vi "Recherche Station FM.vi"() -> ()   [LabVIEW 2013]
uses:
  <vilib>/measure/NI_MAPro.lvlib
  <instrlib>/niUSRP/niUSRP Fetch Rx Data (CDB WDT).vi
  <vilib>/measure/maspectr.llb/FFT Power Spectrum and PSD for 1 Chan (CDB).vi
panel:
  in  "averaging parameters":T1={"averaging mode"=enum."Peak hold", "weighting mode"=enum."Exponential", "number of averages"=10}
  out "IQ Plot":waveform(dbl)[](graph)
  in  "Stop Button":bool
  out "Frequency Plot":cluster{"f0":dbl, "df":dbl, "magnitude":dbl[]}(graph)
  in  "device names":refnum<k15>="192.168.10.2"
  in  "active antenna":string="RX2"
  in  "timeout":dbl=10.0
  in  "number of samples":i64=10000
  out "error out":errorcluster
  out "coerced gain":dbl=10.0 format="%#_6f"
  out "coerced carrier frequency":dbl=315000000.0 format="%#_6p"
  out "coerced IQ rate":dbl=5000000.0 format="%#_6p"
  in  "gain":dbl=10.0 format="%#_6f"
  in  "carrier frequency":dbl=100000000.0 format="%#_6p"
  in  "IQ rate":dbl=4000000.0 format="%#_6p"
  # "IQ Receiver"
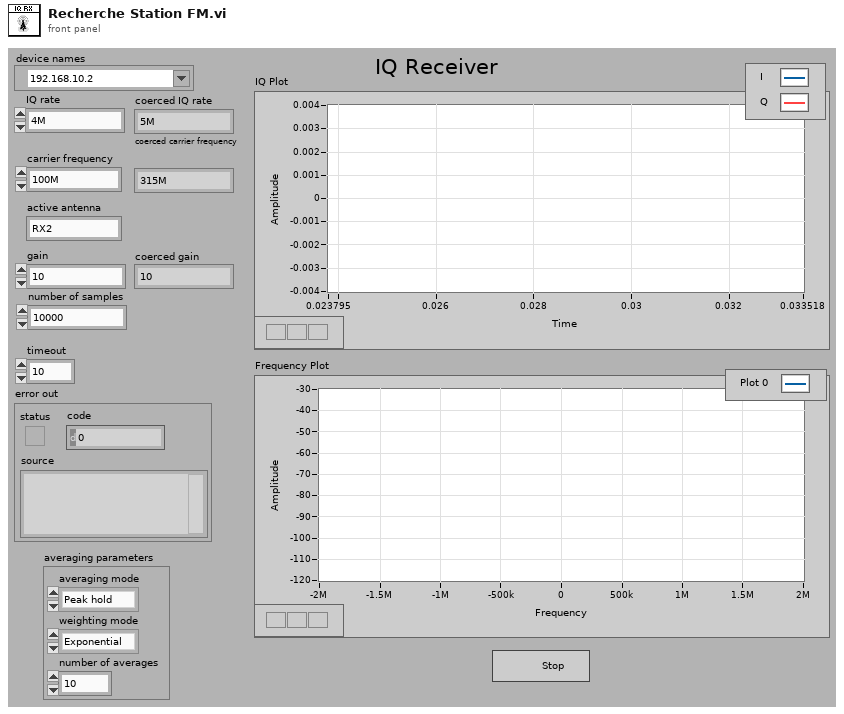
[diagram p1: front panel]
types:
  T1 = cluster{"averaging mode":enum16{"No averaging", "Vector averaging", "RMS averaging", "Peak hold"}, "weighting mode":enum16{"Linear", "Exponential"}, "number of averages":u32}
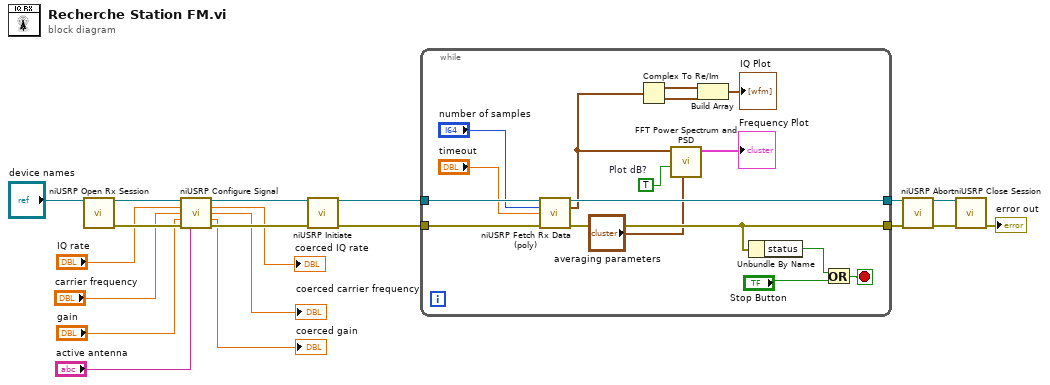
[diagram p0: block diagram]
diagram:
  n1 = call <instrlib>:"niUSRP Open Rx Session.vi"("device names"="device names") -> ("session handle out"=w18:refnum<k15>, "error out"=w17:errorcluster)  [unwired: 13 in]
  n2 = call <instrlib>:"niUSRP Configure Signal.vi"("session handle"=w18, "IQ rate"="IQ rate", "carrier frequency"="carrier frequency", "gain"="gain", "error in (no error)"=w17, "active antenna"="active antenna") -> ("session handle out"=w7:refnum<k15>, "coerced IQ rate"=→"coerced IQ rate":dbl, "coerced carrier frequency"=→"coerced carrier frequency":dbl, "coerced gain"=→"coerced gain":dbl, "error out"=w9:errorcluster)  [unwired: 5 in]
  n3 = call <instrlib>:"niUSRP Initiate.vi"("session handle"=w7, "error in (no error)"=w9) -> ("session handle out"=w13:refnum<k15>, "error out"=w12:errorcluster)  [unwired: 12 in]
  n4 = while {
    tunnel: w13 -> [w35]
    tunnel: w12 -> [w34]
    tunnel: [w29] -> w2
    tunnel: [w28] -> w1
    stop <- w27 stop-if-true
    w30 = TRUE  # Plot dB?
    n5 = call-poly <instrlib>:"niUSRP Fetch Rx Data (poly).vi"("session handle"=w35, "number of samples"="number of samples", "timeout"="timeout", "error in (no error)"=w34) -> ("session handle out"=w29:refnum<k15>, "data"=w21:waveform(cdb), "error out"=w28:errorcluster)  [unwired: 8 in, 1 out]
    n6 = Complex To Re/Im(x + iy=w21) -> (x=w26:waveform(dbl), y=w25:waveform(dbl))
    n7 = call-poly <vilib>:"FFT Power Spectrum and PSD.vi"("averaging parameters"="averaging parameters", "dB On (F)"=w30, "time signal"=w21) -> ("Power Spectrum / PSD"=→"Frequency Plot":cluster{"f0":dbl, "df":dbl, "magnitude":dbl[]})  [unwired: 5 in, 3 out]
    n8 = Build Array(w26, w25) -> (→"IQ Plot":waveform(dbl)[])
    n9 = Unbundle By Name(w28) -> ("status"=w33:bool)
    n10 = Or(x=w33, y="Stop Button") -> (x .or. y?=w27:bool)
  }
  n11 = call <instrlib>:"niUSRP Abort.vi"("session handle"=w2, "error in (no error)"=w1) -> ("session handle out"=w15:refnum<k15>, "error out"=w14:errorcluster)  [unwired: 12 in]
  n12 = call <instrlib>:"niUSRP Close Session.vi"("session handle"=w15, "error in (no error)"=w14) -> ("error out"=→"error out":errorcluster)  [unwired: 13 in]
